vi "Sub V.vi"(9 "VISA resource name":refnum<visa-resource-name>="com4", 10 "升温速度":string) -> ()   [LabVIEW 2021]
uses:
  <vilib>/Instr/_visa.llb/VISA Configure Serial Port (Instr).vi
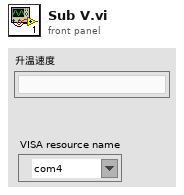
[diagram p1: front panel]
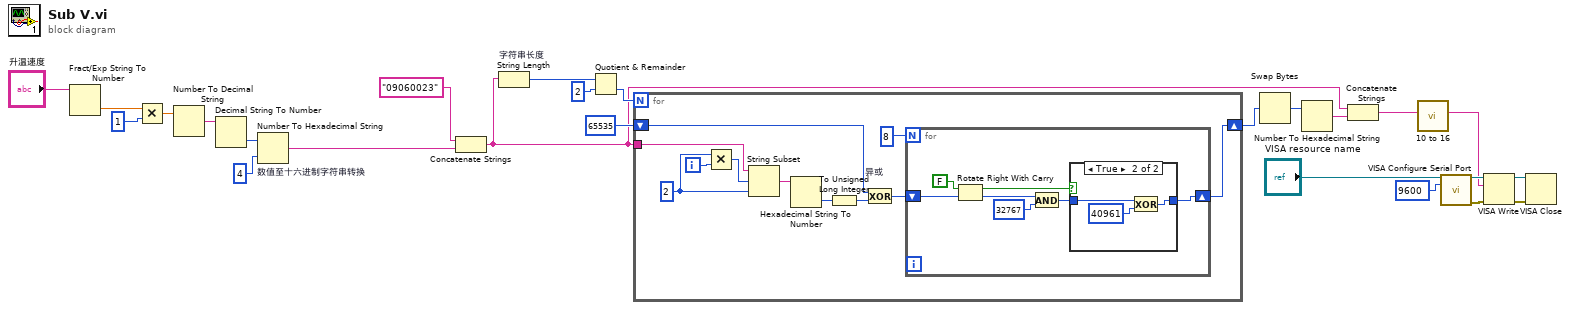
[diagram p0: block diagram]
diagram:
  n1 = Fract/Exp String To Number(string="升温速度") -> (number=w3:dbl)  [unwired: 3 in, 1 out]
  n2 = Multiply(x=w3, y=1) -> (x*y=w2:dbl)
  n3 = Number To Decimal String(number=w2) -> (decimal integer string=w1:string)  [unwired: 1 in]
  n4 = Decimal String To Number(string=w1) -> (number=w22:i32)  [unwired: 2 in, 1 out]
  n5 = Number To Hexadecimal String "数值至十六进制字符串转换"(1:4, 2:w22) -> (0:w23:string)
  n6 = Concatenate Strings("09060023" ("写入缓冲区"), w23) -> (w14:string)
  n7 = String Length "字符串长度"(string=w14) -> (length=w19:i32)
  n8 = Quotient & Remainder(x=w19, y=2) -> (floor(x/y)=w21:i32)  [unwired: 1 out]
  n9 = for {
    N: w21 -> [_]
    tunnel: w14 -> [w36]
    shift-right: [w26] -> w17
    shift-left: 65535 -> [w27]
    i -> [w34]
    w35 = 2
    n10 = Multiply(x=w35, y=w34) -> (x*y=w33:i32)
    n11 = String Subset ("截取字符串")(string=w36, offset (0)=w33, length (rest)=w35) -> (substring=w32:string)
    n12 = Hexadecimal String To Number ("十六进制数字符串至数值转换")(string=w32) -> (number=w31:u32)  [unwired: 2 in, 1 out]
    n13 = To Unsigned Long Integer ("转换为无符号长整型")(number=w31) -> (unsigned 32bit integer=w30:u32)
    n14 = Exclusive Or "异或"(1:w30, 2:w27) -> (0:w28:u32)
    n15 = for {
      N: 8 -> [_]
      shift-right: [w41] -> w26
      shift-left: w28 -> [w43]
      n16 = Rotate Right With Carry(2:w43, 3:FALSE) -> (0:w39:u32, 1:w40:bool)
      n17 = And(x=w39, y=u32 32767) -> (x .and. y?=w38:u32)
      n18 = case shown="True" w40 {
        tunnel: w38 -> [w44 w46]
        tunnel: [w44 w45] -> w41
        frame False {
        }
        frame True {
          n19 = Exclusive Or(1:u32 40961, 2:w46) -> (0:w45:u32)
        }
      }
    }
  }
  n20 = Swap Bytes ("交换字节")(anything=w17) -> (byte swapped=w16:u32)
  n21 = Number To Hexadecimal String ("数值至十六进制字符串转换")(2:w16) -> (0:w15:string)  [unwired: 1 in]
  n22 = Concatenate Strings(w14, w15) -> (w7:string)
  n23 = call "10 to 16.vi"("字符串"=w7) -> ("字符串 2"=w6:string)  [unwired: 10 in]
  n24 = call-poly "VISA Configure Serial Port"("VISA resource name"="VISA resource name", "baud rate (9600)"=u32 9600) -> ("VISA resource name out"=w12:refnum<visa-resource-name>, "error out"=w8:errorcluster)  [unwired: 12 in]
  n25 = VISA Write ("VISA写入")(VISA resource name=w12, write buffer=w6, error in (no error)=w8) -> (VISA resource name out=w10:refnum<visa-resource-name>, error out=w9:errorcluster)  [unwired: 1 out]
  n26 = VISA Close(VISA resource name=w10, error in (no error)=w9) -> ()  [unwired: 1 out]
